vi "Update Data.vi"(7 "NIVS.System Definition Root":refnum<k24>, 8 "Error In":errorcluster, 9 "Indicator?":bool, 10 "Control Reference In":refnum<vi>, 11 "Custom Data Cluster In":T1) -> (0 "error Out":errorcluster, 3 "Custom Data Cluster Out":T1)   [LabVIEW 2011]
doc: "This VI prompts the user to select a channel. Once a channel is selected, it is either added to the array of 'paths' and 'indices' OR if it has already been assigned a channel before, then it is indexed and the Path is overwritten."
uses:
  Custom Data Cluster Control.ctl
  NationalInstruments.VeriStand.SystemStorage
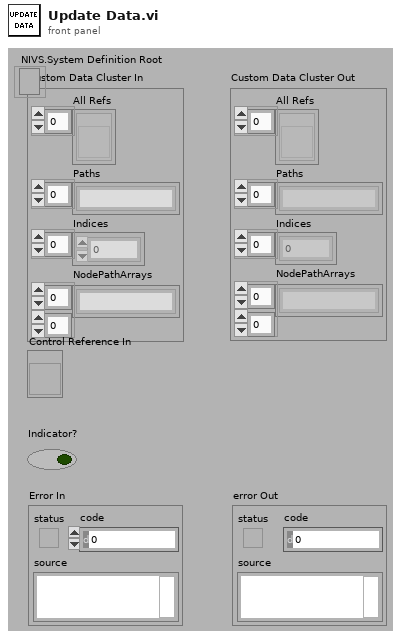
[diagram p1: front panel]
types:
  T1 = typedef "Custom Data Cluster Control.ctl" = cluster{"All Refs":refnum<vi>[], "Paths":string[], "Indices":u32[], "NodePathArrays":string[][]}
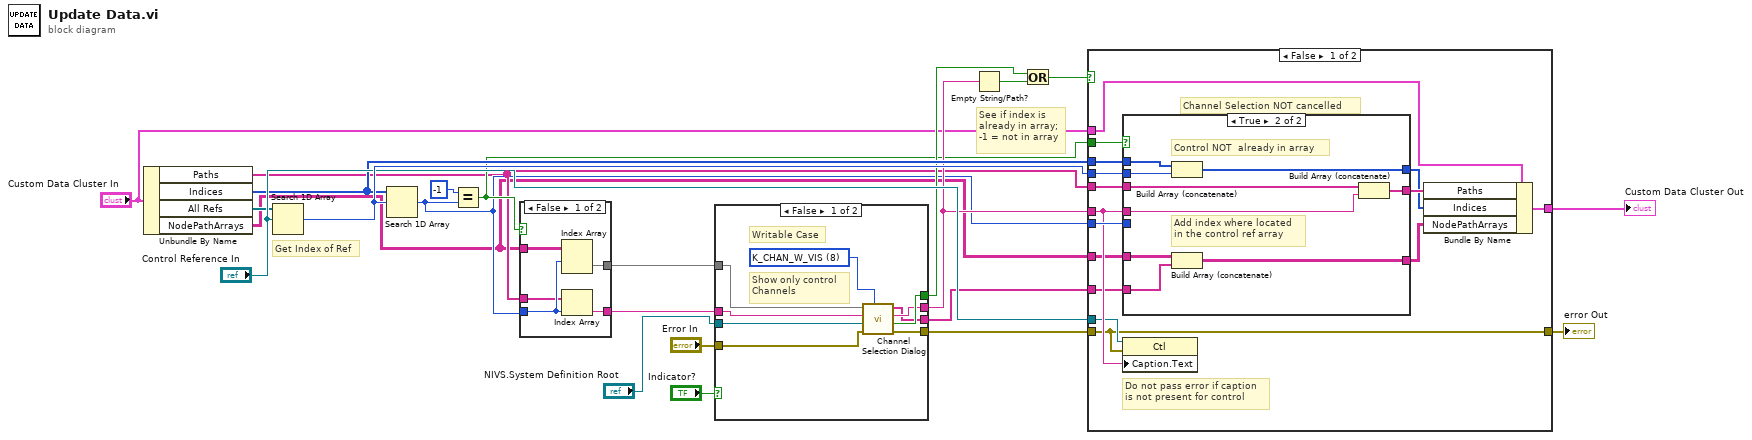
[diagram p0: block diagram]
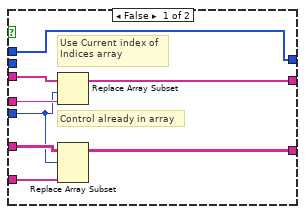
[diagram p3: hidden frame]
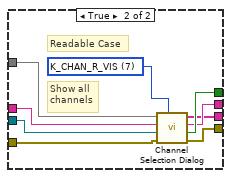
[diagram p5: hidden frame]
diagram:
  # "See if index is\nalready in array;\n-1 = not in array"
  # "Get Index of Ref"
  n1 = Unbundle By Name("Custom Data Cluster In") -> ("Paths"=w3:string[], "Indices"=w17:u32[], "All Refs"=w16:refnum<vi>[], "NodePathArrays"=w2:string[][])
  n2 = Search 1D Array(1D array=w16, element="Control Reference In") -> (index of element=w20:i32)  [unwired: 1 in]
  n3 = Search 1D Array(1D array=w17, element=w20) -> (index of element=w6:i32)  [unwired: 1 in]
  n4 = Equal?(x=-1 ("index of element"), y=w6) -> (x = y?=w8:bool)
  n5 = case shown="False" w8 {
    tunnel: w6 -> [w26 _]
    tunnel: [w28 _] -> w5
    tunnel: [w27 _] -> w4
    tunnel: w2 -> [w25 _]
    tunnel: w3 -> [w24 _]
    frame False {
      n6 = Index Array(array=w25, index (row)=w26) -> (element=w28:string[])  [unwired: 1 in]
      n7 = Index Array(array=w24, index=w26) -> (element=w27:string)
    }
    frame True {
    }
  }
  n8 = case shown="False" "Indicator?" {
    tunnel: [w34 w42] -> w15
    tunnel: [w33 w41] -> w12
    tunnel: "NIVS.System Definition Root" -> [w35 w45]
    tunnel: "Error In" -> [w37 w44]
    tunnel: [w36 w43] -> w9
    tunnel: w5 -> [w32 w40]
    tunnel: w4 -> [w31 w39]
    tunnel: [w29 w38] -> w1
    frame False {
      w30 = u8 8 items=["K_CHAN_R", "K_CHAN_W", "K_CHAN_RW", "K_CHAN_VOLT", "K_CHAN_FAULT", "K_ALL", "K_CUSTOM", "K_CHAN_R_VIS", "K_CHAN_W_VIS", "K_CHAN_RW_VIS", "K_CHAN_VOLT_VIS", "K_CHAN_FAULT_VIS"] ("DisplayFilter")
      # "Writable Case"
      # "Show only control\nChannels"
      n9 = call "Channel Selection Dialog.vi"("DisplayFilter"=w30, "error in (no error)"=w37, "NIVS.System Definition Root"=w35, "Start NodePath"=w31, "Start NodePathArray"=w32) -> ("error out"=w36:errorcluster, "Cancelled?"=w34:bool, "Selected NodePath"=w33:string, "Selected NodePathArray"=w29:string[])  [unwired: 3 in]
    }
    frame True {
      w46 = u8 7 items=["K_CHAN_R", "K_CHAN_W", "K_CHAN_RW", "K_CHAN_VOLT", "K_CHAN_FAULT", "K_ALL", "K_CUSTOM", "K_CHAN_R_VIS", "K_CHAN_W_VIS", "K_CHAN_RW_VIS", "K_CHAN_VOLT_VIS", "K_CHAN_FAULT_VIS"] ("DisplayFilter")
      # "Readable Case"
      # "Show all\nchannels"
      n10 = call "Channel Selection Dialog.vi"("DisplayFilter"=w46, "error in (no error)"=w44, "NIVS.System Definition Root"=w45, "Start NodePath"=w39, "Start NodePathArray"=w40) -> ("error out"=w43:errorcluster, "Cancelled?"=w42:bool, "Selected NodePath"=w41:string, "Selected NodePathArray"=w38:string[])  [unwired: 3 in]
    }
  }
  n11 = Empty String/Path?(string/path=w12) -> (empty?=w14:bool)
  n12 = Or(x=w15, y=w14) -> (x .or. y?=w13:bool)
  n13 = case shown="False" w13 {
    tunnel: "Custom Data Cluster In" -> [w56 w80]
    tunnel: w3 -> [w61 _]
    tunnel: w17 -> [w59 _]
    tunnel: w20 -> [w60 _]
    tunnel: w12 -> [w52 _]
    tunnel: [w55 w80] -> w22
    tunnel: w8 -> [w54 _]
    tunnel: w6 -> [w53 _]
    tunnel: "Control Reference In" -> [w51 _]
    tunnel: w9 -> [w50 w79]
    tunnel: [w50 w79] -> w18
    tunnel: w2 -> [w48 _]
    tunnel: w1 -> [w47 _]
    frame False {
      # "Do not pass error if caption\nis not present for control"
      # "Channel Selection NOT cancelled"
      n14 = case shown="True" w54 {
        tunnel: w61 -> [w67 w77]
        tunnel: w52 -> [w69 w76]
        tunnel: w60 -> [_ w73]
        tunnel: w59 -> [w68 w78]
        tunnel: [w68 w74] -> w57
        tunnel: [w66 w75] -> w58
        tunnel: w53 -> [w63 _]
        tunnel: [w64 w72] -> w49
        tunnel: w48 -> [w65 w71]
        tunnel: w47 -> [w62 w70]
        frame False {
          # "Use Current index of\nIndices array"
          # "Control already in array"
          n15 = Replace Array Subset(array=w67, new element=w69, index=w63) -> (w66:string[])
          n16 = Replace Array Subset(array=w65, new element=w62, index (row)=w63) -> (w64:string[][])  [unwired: 1 in]
        }
        frame True {
          # "Add index where located\nin the control ref array"
          # "Control NOT  already in array"
          n17 = Build Array (concatenate)(w78, w73) -> (w74:u32[])
          n18 = Build Array (concatenate)(w71, w70) -> (w72:string[][])
          n19 = Build Array (concatenate)(w77, w76) -> (w75:string[])
        }
      }
      n20 = property class="Ctl"(reference=w51, error in=w50, "Caption.Text"=w52) -> ()  [unwired: 2 out]
      n21 = Bundle By Name(cluster=w56, "Paths"=w58, "Indices"=w57, "NodePathArrays"=w49) -> (w55:T1)
    }
    frame True {
      # "Cancelled = True; Change nothing"
    }
  }
  "Custom Data Cluster Out" <- w22
  "error Out" <- w18
